vi "JAVA_DriveType.vi"() -> ()   [LabVIEW 2016]
uses:
  TypeDef/ENUM_Drive_Type Select.ctl
panel:
  in  "Drive Type":T1
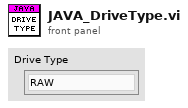
[diagram p1: front panel]
types:
  T1 = typedef "ENUM_Drive_Type Select.ctl" = enum16{"RAW", "CHEESY", "FULL_BRAKE", "MAGIC", "AUTO_GEAR_DROP", "PATH"}
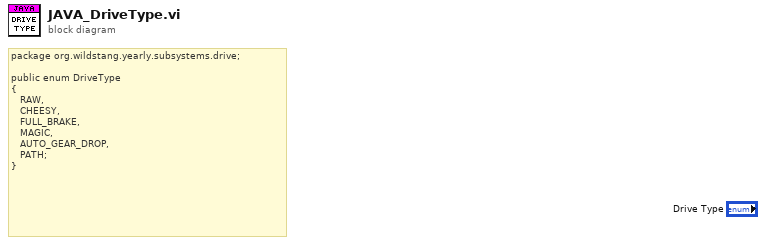
[diagram p0: block diagram]
diagram:
  # "package org.wildstang.yearly.subsystems.drive;\n\npublic enum DriveType\n{\n   RAW,\n   CHEESY,\n   FULL_BRAKE,\n   MAGIC,\n   AUTO_GEAR_DROP,\n   PATH;\n}"
